vi "RREQ_Packet_Encode_and_Decode_Test.vi"() -> ()   [LabVIEW 2017]
uses:
  Classes/ADCP.lvclass
panel:
  out "RREQ out":T1
  in  "RREQ_Packet In":T1
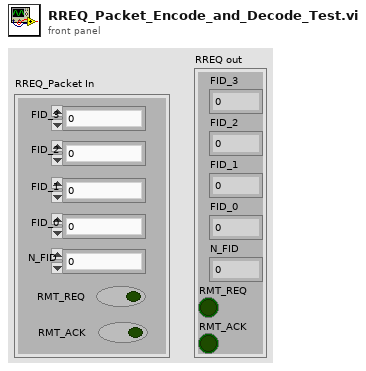
[diagram p1: front panel]
types:
  T1 = cluster{"FID_3":u8, "FID_2":u8, "FID_1":u8, "FID_0":u8, "N_FID":u8, "RMT_REQ":bool, "RMT_ACK":bool}
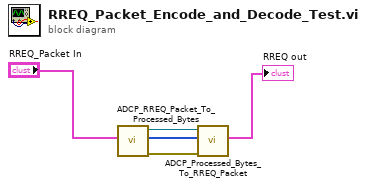
[diagram p0: block diagram]
diagram:
  n1 = call "ADCP_RREQ_Packet_To_Processed_Bytes.vi"("RREQ_Packet"="RREQ_Packet In") -> ("error out"=w2:errorcluster, "Processed Packet Bytes"=w3:u8[], "ADCP Out"=w4:refnum<class "ADCP.lvclass">)  [unwired: 8 in]
  n2 = call "ADCP_Processed_Bytes_To_RREQ_Packet.vi"("error in (no error)"=w2, "Processed Packet Bytes"=w3, "ADCP In"=w4) -> ("RREQ out"=→"RREQ out":T1)  [unwired: 6 in, 2 out]
